vi "IleCzasu.vi"() -> ()   [LabVIEW 2024]
uses:
  StoperEnum.ctl
panel:
  out "time (s)":dbl format="%#.3g"
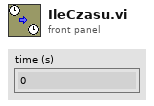
[diagram p1: front panel]
types:
  T1 = typedef "StoperEnum.ctl" = enum16{"Start", "Time"}
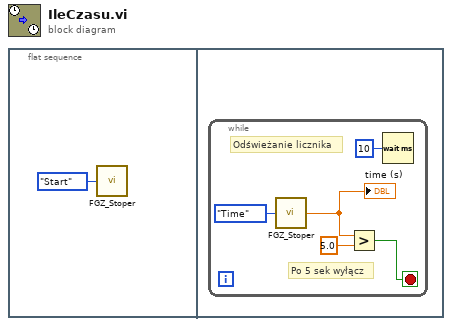
[diagram p0: block diagram]
diagram:
  n1 = flat-sequence {
    frame #0 {
      n2 = call "FGZ_Stoper.vi"("StoperEnum"=StoperEnum."Start") -> ()  [unwired: 4 in, 1 out]
    }
    frame #1 {
      n3 = while {
        stop <- w3 stop-if-true
        # "Po 5 sek wyłącz"
        # "Odświeżanie licznika"
        n4 = call "FGZ_Stoper.vi"("StoperEnum"=StoperEnum."Time") -> ("time (s)"=w4:dbl)  [unwired: 4 in]
        "time (s)" <- w4
        n5 = Greater?(x=w4, y=5.0) -> (0:w3:bool)
        n6 = Wait (ms)(milliseconds to wait=u32 10) -> ()  [unwired: 1 out]
      }
    }
  }
